vi "ReadActor.vi"(7 "ConcreteActor":refnum<class "ConcreteActor.lvclass">) -> (3 "Actor":refnum<class "Actor.lvclass">)   [LabVIEW 2020, in "_Template.lvlib" / "ActorTemplate.lvlib" / "{{Name}}.lvlib" / "ConcreteActor.lvclass"]
uses:
  ConcreteActor.lvclass
  jettl/jettl/Actor/Actor.lvclass
  ConcreteActor.lvclass/ConcreteActor.ctl
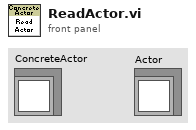
[diagram p1: front panel]
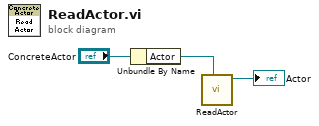
[diagram p0: block diagram]
diagram:
  n1 = Unbundle By Name("ConcreteActor") -> ("Actor"=w2:refnum<class "Actor.lvclass">)
  n2 = call-dynamic "ReadActor.vi"("Actor"=w2) -> ("Actor"=→"Actor":refnum<class "Actor.lvclass">)  [unwired: 10 in]
